vi "Add Scan Engine Custom Device and Return Slots.vi"(8 "error in":errorcluster, 11 "target ref in":refnum<k39>) -> (0 "error out":errorcluster, 2 "slot refs":T1[](array[typedef]) format="%.0x", 3 "target ref out":refnum<k39>)   [LabVIEW 2020, in "Scan Engine Scripting API Custom Device Unit Tests.lvclass"]
uses:
  Scan Engine Scripting API Custom Device Unit Tests.lvclass
  Scan Engine Scripting API Custom Device Unit Tests.lvclass/Scan Engine Scripting API Custom Device Unit Tests.ctl
  Scripting/Scan Engine Scripting.lvlib
  Shared/Type Defs/Main Settings.ctl
  Shared/SEECD Shared.lvlib
  Shared/Type Defs/Local Chassis Settings.ctl
  <vilib>/NI VeriStand/Custom Device API/Custom Device Item Ref.ctl
  <vilib>/NI VeriStand/Custom Device API/Custom Device API.lvlib
  C:/Users/Administrator/Desktop/Jatin/All DNC DLLs/NationalInstruments.VeriStand.SystemDefinitionAPI.dll
  Jatin/All DNC DLLs/NationalInstruments.VeriStand.SystemDefinitionAPI.dll
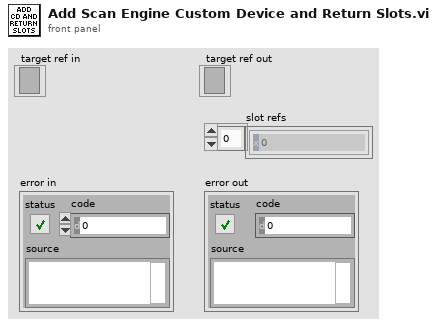
[diagram p1: front panel]
types:
  T1 = typedef "Custom Device API.lvlib/Custom Device Item Ref.ctl" = u64
  T2 = typedef "SEECD Shared.lvlib/Local Chassis Settings.ctl" = cluster{"name":string, "number of slots":i32}
  T3 = typedef "SEECD Shared.lvlib/Main Settings.ctl" = cluster{"sync to scan":bool, "scan engine decimation":u16, "delay after FPGA load (s)":u16}
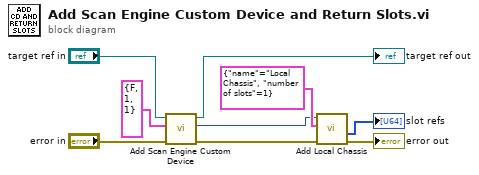
[diagram p0: block diagram]
diagram:
  n1 = call "Add Scan Engine Custom Device.vi"("error in"="error in", "settings"=T3 {"sync to scan"=FALSE, "scan engine decimation"=1, "delay after FPGA load (s)"=1}, "NationalInstruments.VeriStand.SystemDefinitionAPI.Target"="target ref in") -> ("error out"=w4:errorcluster, "scan engine custom device ref"=w5:T1, "NationalInstruments.VeriStand.SystemDefinitionAPI.Target"=→"target ref out":refnum<k39>)  [unwired: 6 in]
  n2 = call "Add Local Chassis.vi"("error in"=w4, "settings"=T2 {"name"="Local Chassis", "number of slots"=1}, "scan engine custom device ref in"=w5) -> ("error out"=→"error out":errorcluster, "slot refs"=→"slot refs":T1[])  [unwired: 4 in, 3 out]
